vi "Main.vi"(11 "Module Admin":refnum<class "Delacor_lib_QMH_Module Admin.lvclass">) -> ()   [LabVIEW 2025, in "Dashboard.lvlib"]
doc: "This template is based off of the Queued Message Handler design pattern and the Queued Message Handler project template that ships with LabVIEW.\n\nThe main difference is that the queue is private to this module and communication between modules is performed via Broadcast and Request events.\n\nRequest events are wrapped in public API methods and are handled in the Event Handling Loop (EHL) of this VI. Any module can register for Broadcast events sent by this module. The EHL generates messages based on user interface actions.\n\nThe Message Handling Loop (MHL) processes messages generated by the EHL, or by other messages. The messages are string values, so new messages can be added easily to the Message Cases case structure in the MHL. Each message cluster can also provide an optional value for Message Data, which is a variant that can be converted to whatever message-specific data is required.\n_____\nBased on DQMH Dev Tools: Project Template 7.1.2.1547."
uses:
  Dashboard.lvlib
  <vilib>/Delacor/Delacor QMH/Libraries/Module Admin_class/Delacor_lib_QMH_Module Admin.lvclass
  OpCore/SQLite/SQLite.lvclass
  <vilib>/Delacor/Delacor QMH/Libraries/Message Queue_class/Delacor_lib_QMH_Message Queue.lvclass/Delacor_lib_QMH_Message Queue.ctl
  <vilib>/Delacor/Delacor QMH/Libraries/Module Admin_class/Delacor_lib_QMH_Module Admin.lvclass/Delacor_lib_QMH_Module Admin.ctl
  <vilib>/Delacor/Delacor QMH/Libraries/Message Queue_class/Delacor_lib_QMH_Message Queue.lvclass
  Module Data--cluster.ctl
  <vilib>/Utility/miscctls.llb/LVPointTypeDef.ctl
  <vilib>/Delacor/Delacor QMH/Libraries/Message Queue_class/Delacor_lib_QMH_Enqueue Message (Single).vi
  Stop Argument--cluster.ctl
  OpCore/OpCore Types/BaselineMode.ctl
  OpCore/OpCore Types/OpCore Types.lvlib
  OpCore/OpCore Types/Baseline Config.ctl
  OpCore/OpCore Types/ShutdownReason.ctl
  OpCore/OpCore Types/SyncDirection.ctl
  OpCore/OpCore Types/TableOverride.ctl
  OpCore/OpCore Types/StationConfig.ctl
  OpCore/Libraries/Connection Monitor/Connection Monitor.lvlib
  OpCore/Libraries/Inbound Sync/Inbound Sync.lvlib
  OpCore/Libraries/Outbound Sync/Outbound Sync.lvlib
  OpCore/Libraries/Connection Monitor/Database Status.ctl
  OpCore/PostgreSQL/PostgreSQL.lvclass
  Launch Modules Argument--cluster.ctl
  OpCore/OpCore Types/CycleDirection.ctl
  OpCore/OpCore Types/CycleStatus.ctl
  OpCore/OpCore Types/SyncCycleResult.ctl
panel:
  in  "Start":bool
  out "Time Stamp":timestamp
  out "Connected":bool
  out "Online":bool
  in  "Force In Sync":bool
  out "Halt?":bool
  out "Last In Sync Results":T1
  out "Last Out Sync Results":T1
  in  "Force Out Sync":bool
  in  "Start Sync":bool
  in  "stop":bool
  out "Schema Version":string
  out "Station ID":string
  out "error out":errorcluster
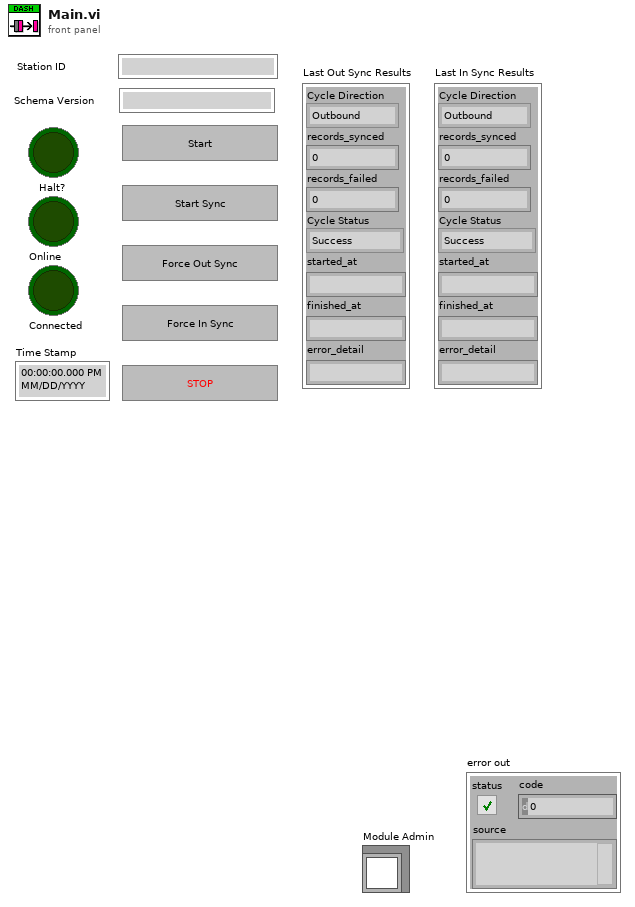
[diagram p1: front panel]
types:
  T1 = typedef "OpCore Types.lvlib/SyncCycleResult.ctl" = cluster{"Cycle Direction":T2, "records_synced":i32, "records_failed":i32, "Cycle Status":T3, "started_at":string, "finished_at":string, "error_detail":string}
  T2 = typedef "OpCore Types.lvlib/CycleDirection.ctl" = enum16{"Outbound", "Inbound", "Startup", "Shutdown", "Baseline", "Provision", "Migration", "Config"}
  T3 = typedef "OpCore Types.lvlib/CycleStatus.ctl" = enum16{"Success", "Partial", "Failed"}
  T4 = typedef "Connection Monitor.lvlib/Broadcast Events--cluster.ctl" = cluster{"Module Did Init":refnum<user-event>, "Status Updated":refnum<user-event>, "Error Reported":refnum<user-event>, "Module Did Stop":refnum<user-event>, "Update Module Execution Status":refnum<user-event>, "Database Online":refnum<user-event>, "Database Offline":refnum<user-event>, "Database Status Updated":refnum<user-event>}
  T5 = typedef "Outbound Sync.lvlib/Broadcast Events--cluster.ctl" = cluster{"Module Did Init":refnum<user-event>, "Status Updated":refnum<user-event>, "Error Reported":refnum<user-event>, "Module Did Stop":refnum<user-event>, "Update Module Execution Status":refnum<user-event>, "Sync Completed":refnum<user-event>}
  T6 = typedef "Inbound Sync.lvlib/Broadcast Events--cluster.ctl" = cluster{"Module Did Init":refnum<user-event>, "Status Updated":refnum<user-event>, "Error Reported":refnum<user-event>, "Module Did Stop":refnum<user-event>, "Update Module Execution Status":refnum<user-event>, "Sync Completed":refnum<user-event>}
  T7 = typedef "Dashboard.lvlib/Request Events--cluster.ctl" = cluster{"Stop Module":refnum<user-event>, "Show Panel":refnum<user-event>, "Hide Panel":refnum<user-event>, "Get Module Execution Status":refnum<user-event>, "Show Diagram":refnum<user-event>, "Private.Launch Modules":refnum<user-event>}
  T8 = typedef "Dashboard.lvlib/Module Data--cluster.ctl" = cluster{"Status":string, "SQLite":refnum<class "SQLite.lvclass">, "StationConfig":T9, "OB Module ID":i32, "IB Module ID":i32, "is online":bool, "CM alive?":bool, "OB alive?":bool, "IB alive?":bool, "IB first cycle seen?":bool, "OB first cycle seen?":bool, "shutting down?":bool, "exit code":i32, "status":bool, "code":i32, "source":string, "ShutdownReason":T12, "OB last cycle at":timestamp, "IB last cycle at":timestamp, "Baseline Config":T13}
  T9 = typedef "OpCore Types.lvlib/StationConfig.ctl" = cluster{"station_id":string, "schema_version":string, "sqlite_path":string, "syncagent_db_path":string, "postgres_conn":string, "sync_interval_sec":i32, "inbound_offset_sec":i32, "batch_size":i32, "table_overrides":T10[]}
  T10 = typedef "OpCore Types.lvlib/TableOverride.ctl" = cluster{"table_name":string, "Sync Direction":T11}
  T11 = typedef "OpCore Types.lvlib/SyncDirection.ctl" = enum16{"Both", "Outbound_Only", "Inbound_Only", "Exclude"}
  T12 = typedef "OpCore Types.lvlib/ShutdownReason.ctl" = enum16{"None", "Operator", "Service", "ModuleDied", "Fatal"}
  T13 = typedef "OpCore Types.lvlib/Baseline Config.ctl" = cluster{"Baseline Mode":T14, "From Date":string, "Chunk Size":i32, "Verify Checksums":bool}
  T14 = typedef "OpCore Types.lvlib/BaselineMode.ctl" = enum16{"None", "Full", "From Date"}
  T15 = enum32{"invalid lock state", "Not Locked", "Locked (No Password)", "Password-protected"}
  T16 = typedef "Dashboard.lvlib/Stop Argument--cluster.ctl" = cluster{"Origin":string, "Exit via Stop Module Req?":bool, "Wait for Module to stop?":bool}
  T17 = typedef "Connection Monitor.lvlib/Database Status.ctl" = cluster{"Time Stamp":timestamp, "isOnline?":bool}
  T18 = typedef "Dashboard.lvlib/Launch Modules Argument--cluster.ctl" = cluster{"OB Module ID":i32, "IB Module ID":i32}
  T19 = typedef "LVPointTypeDef.ctl" = cluster{"Horizontal":i16, "Vertical":i16}
  T20 = enum32{"Invalid", "Standard", "Closed", "Hidden", "Minimized", "Maximized"}
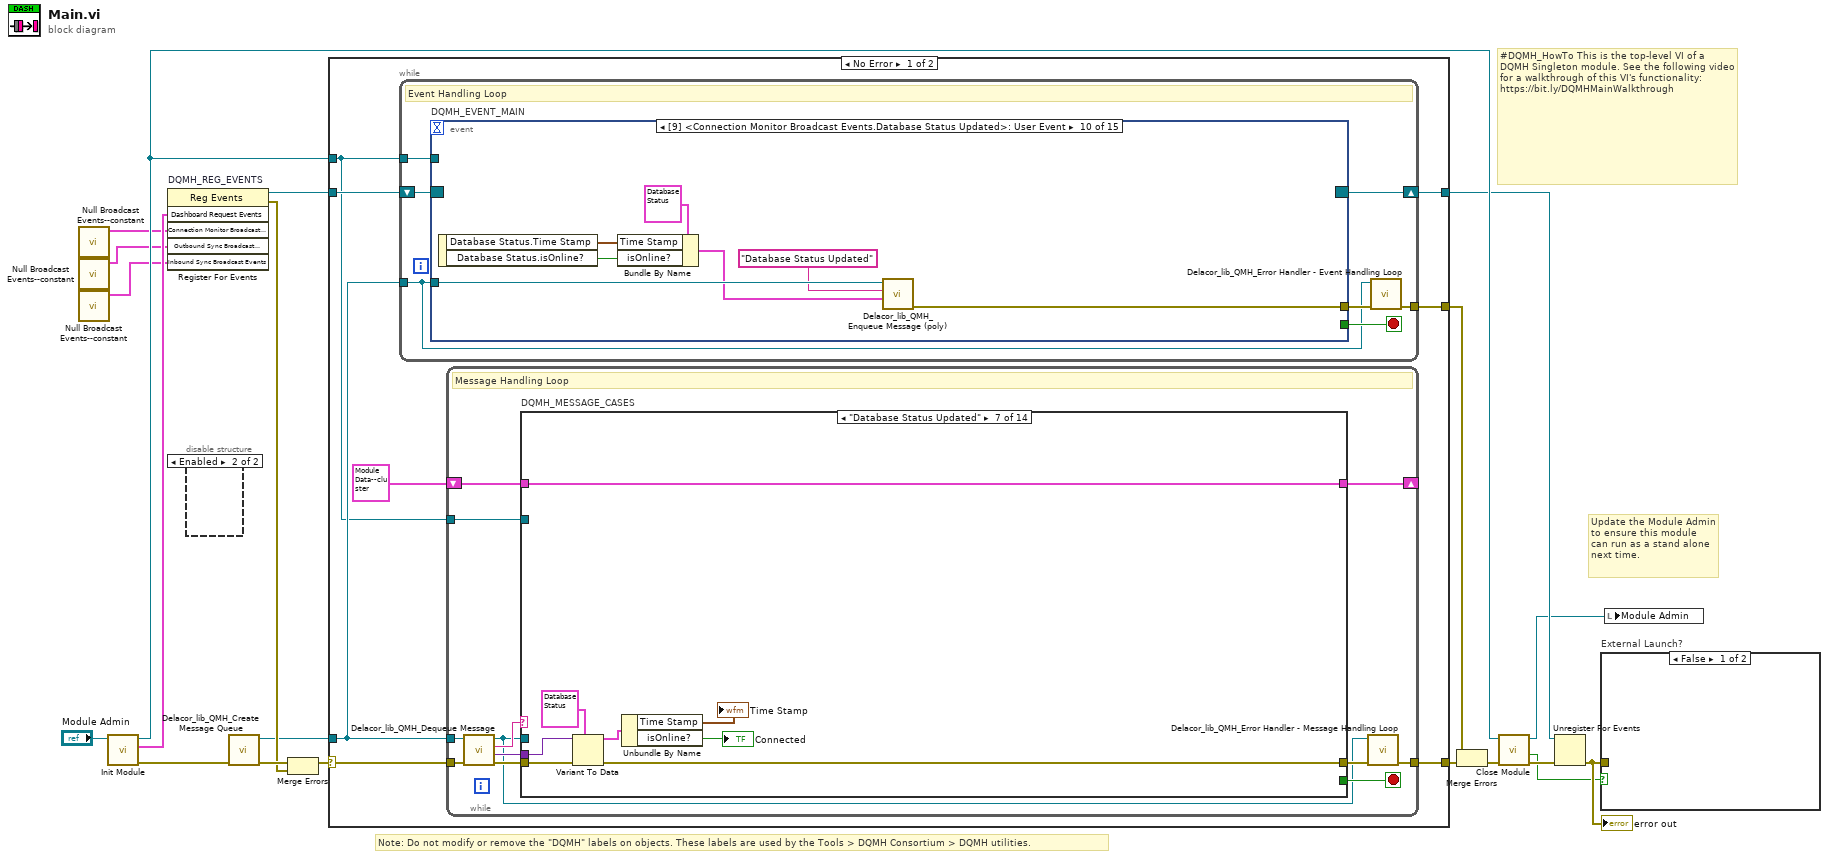
[diagram p0: block diagram]
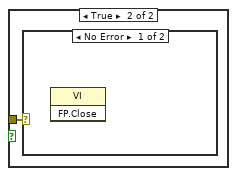
[diagram p3: hidden frame]
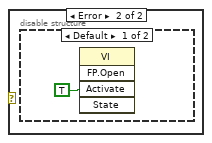
[diagram p4: hidden frame]
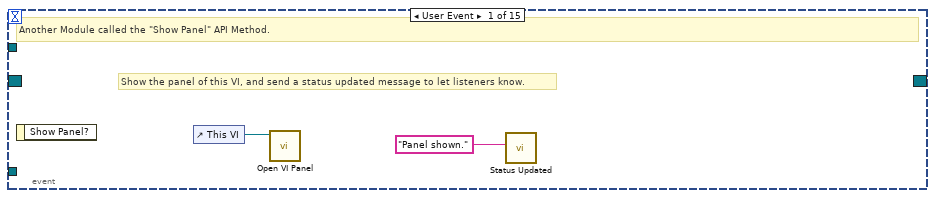
[diagram p6: hidden frame]
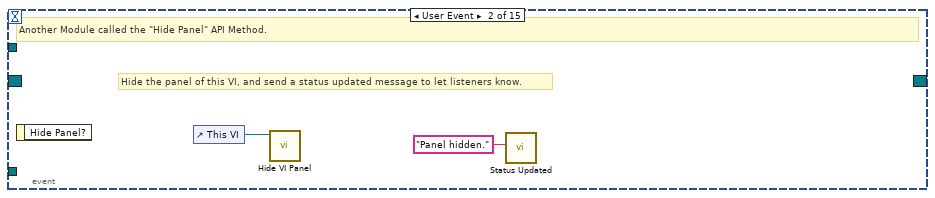
[diagram p7: hidden frame]
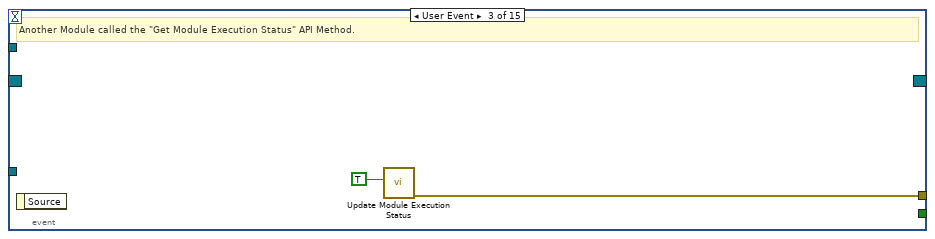
[diagram p8: hidden frame]
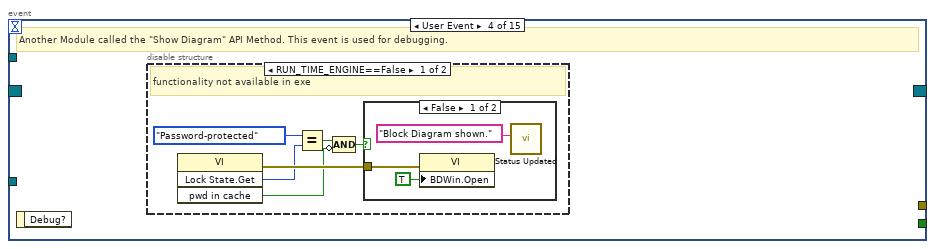
[diagram p9: hidden frame]
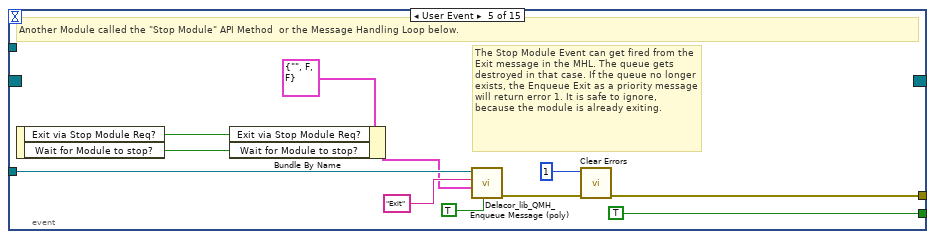
[diagram p12: hidden frame]
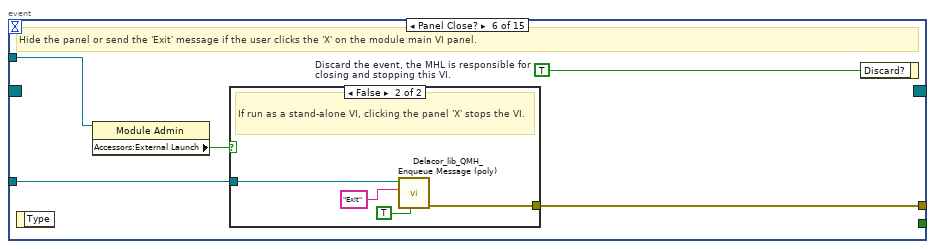
[diagram p13: hidden frame]
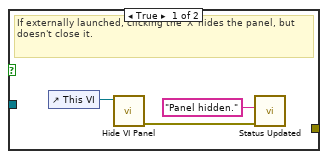
[diagram p14: hidden frame]
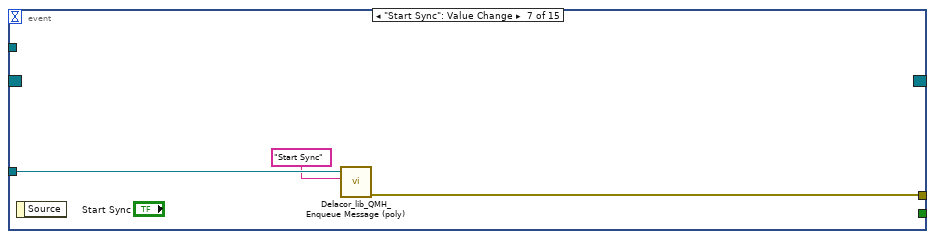
[diagram p15: hidden frame]
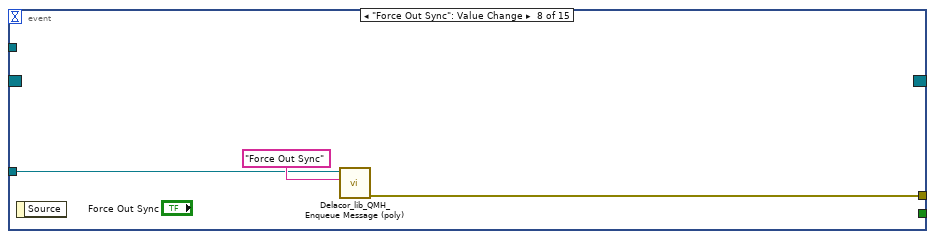
[diagram p16: hidden frame]
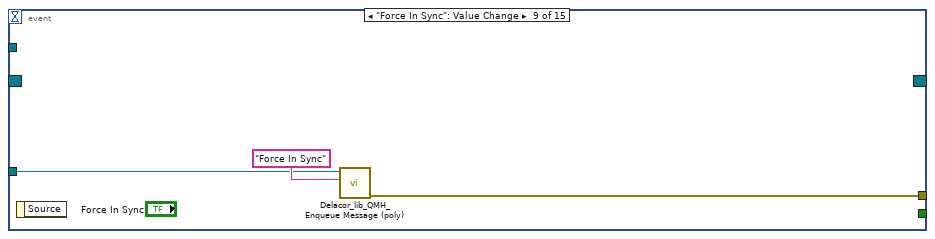
[diagram p17: hidden frame]
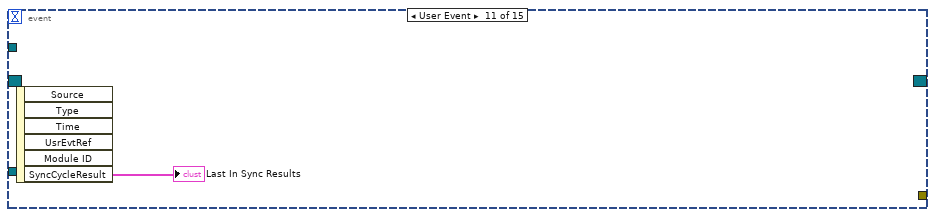
[diagram p18: hidden frame]
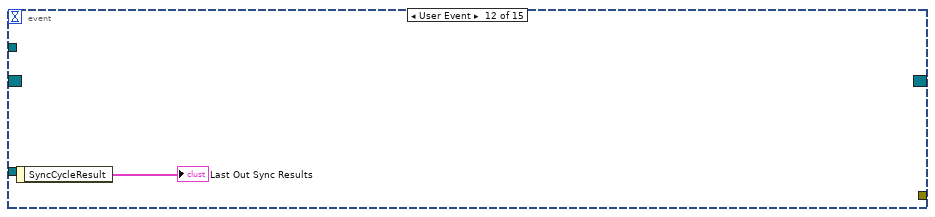
[diagram p19: hidden frame]
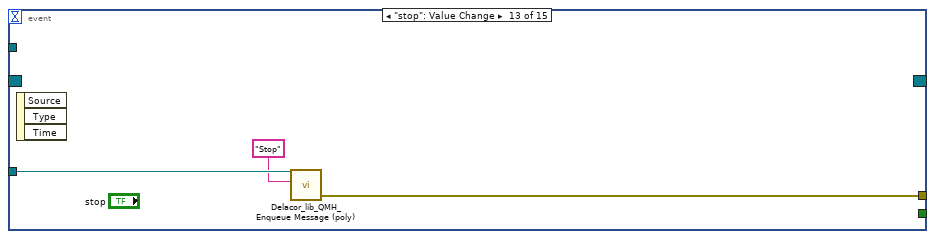
[diagram p20: hidden frame]
diagram:
  # "#DQMH_HowTo This is the top-level VI of a DQMH Singleton module. See the following video for a walkthrough of this VI's functionality: https://bit.ly/DQMHMainWalkthrough"
  # "Note: Do not modify or remove the \"DQMH\" labels on objects. These labels are used by the Tools > DQMH Consortium > DQMH utilities."
  # "Update the Module Admin to ensure this module can run as a stand alone next time."
  n1 = call "Null Broadcast Events--constant.vi"() -> ("Connection Monitor Broadcast Events"=w3:T4)  [unwired: 11 in]
  n2 = call "Null Broadcast Events--constant.vi"() -> ("Outbound Sync Broadcast Events"=w2:T5)  [unwired: 11 in]
  n3 = call "Null Broadcast Events--constant.vi"() -> ("Inbound Sync Broadcast Events"=w1:T6)  [unwired: 11 in]
  n4 = call "Init Module.vi"("Singleton Module Admin in"="Module Admin") -> ("error out"=w19:errorcluster, "Dashboard Request Events"=w8:T7, "Singleton Module Admin out"=w11:refnum<class "Delacor_lib_QMH_Module Admin.lvclass">)  [unwired: 8 in]
  n5 = register-events "DQMH_REG_EVENTS"(w8, w3, w2, w1) -> (reference out=w9:refnum<event-registration>, error out=w12:errorcluster)  [unwired: 2 in]
  n6 = disable-structure shown="Enabled" {
    frame Disabled {
    }
    frame Enabled {
    }
  }
  n7 = call <vilib>:"Delacor_lib_QMH_Create Message Queue.vi"("error in"=w19) -> ("error out"=w14:errorcluster, "Message Queue"=w7:refnum<class "Delacor_lib_QMH_Message Queue.lvclass">)  [unwired: 9 in]
  n8 = Merge Errors(w14, w12) -> (w13:errorcluster)
  n9 = case shown="No Error" w13 {
    selector: w13 -> [w26 w268]
    tunnel: [w28 w267] -> w20
    tunnel: [w25 w266] -> w10
    tunnel: w9 -> [w23 w266]
    tunnel: w7 -> [w22 w261]
    tunnel: [w27 _] -> w17
    tunnel: w11 -> [w21 w262]
    frame No Error {
      n10 = while {
        tunnel: w22 -> [w29]
        shift-right: [w32] -> w25
        shift-left: w23 -> [w33]
        tunnel: [w34] -> w27
        tunnel: w21 -> [w30]
        stop <- w31 stop-if-true
        # "Event Handling Loop"
        n11 = event "DQMH_EVENT_MAIN" shown="[9] <Connection Monitor Broadcast Events.Database Status Updated>: User Event" {
          selector: w33 -> [_ _ _ _ _ _ _ _ _ _ _ _ _ _ w110]
          dyn-events: [_ _ _ _ _ _ _ _ _ _ _ _ _ _ w106] -> w32
          timeout: _ -> [_ _ _ _ _ _ _ _ _ _ _ _ _ _ _]
          tunnel: [_ _ _ _ TRUE ("Discard?") _ _ _ _ _ _ _ _ _ _] -> w31
          tunnel: w29 -> [_ _ _ _ w57 w64 w76 w77 w80 w89 _ _ w94 w101 _]
          tunnel: [_ _ w41 _ w60 w66 w74 w78 w81 w88 _ _ w93 w95 w102] -> w35
          tunnel: w30 -> [_ _ _ _ _ w63 _ _ _ _ _ _ _ _ _]
          event User Event {
            # "Show the panel of this VI, and send a status updated message to let listeners know."
            # "Another Module called the \"Show Panel\" API Method."
            n12 = event-data() -> ()  [unwired: 1 in, 1 out]
            n13 = control-ref of="This VI"() -> (w37:refnum<vi>)
            n14 = call "Open VI Panel.vi"("VI"=w37) -> ()  [unwired: 10 in, 1 out]
            n15 = call "Status Updated.vi"("Status"="Panel shown." ("format string")) -> ()  [unwired: 10 in, 1 out]
          }
          event User Event {
            # "Hide the panel of this VI, and send a status updated message to let listeners know."
            # "Another Module called the \"Hide Panel\" API Method."
            n16 = event-data() -> ()  [unwired: 1 in, 1 out]
            n17 = control-ref of="This VI"() -> (w39:refnum<vi>)
            n18 = call "Hide VI Panel.vi"("VI"=w39) -> ()  [unwired: 10 in, 1 out]
            n19 = call "Status Updated.vi"("Status"="Panel hidden." ("format string")) -> ()  [unwired: 10 in, 1 out]
          }
          event User Event {
            # "Another Module called the \"Get Module Execution Status\" API Method."
            n20 = event-data() -> ()  [unwired: 1 in, 1 out]
            n21 = call "Update Module Execution Status.vi"("Running?"=TRUE) -> ("error out"=w41:errorcluster)  [unwired: 10 in]
          }
          event User Event {
            # "Another Module called the \"Show Diagram\" API Method. This event is used for debugging."
            n22 = event-data() -> ()  [unwired: 1 in, 1 out]
            n23 = disable-structure shown="RUN_TIME_ENGINE==False" {
              frame condition #0 (active) {
                # "functionality not available in exe"
                n24 = invoke on="Invoke Node" class="VI" method="Lock State.Get"() -> (error out=w47:errorcluster, "Get Lock State"=w46:T15, "pwd in cache"=w43:bool)  [unwired: 4 in, 1 out]
                n25 = Equal?(x=T15."Password-protected", y=w46) -> (x = y?=w44:bool)
                n26 = Compound Arithmetic op=AND(w44, invert w43) -> (w42:bool)
                n27 = case shown="False" w42 {
                  tunnel: w47 -> [w50 _]
                  frame False {
                    n28 = property on="Property Node" class="VI"(error in=w50, "BDWin.Open"=TRUE ("Block Diagram Window:Open")) -> ()  [unwired: 1 in, 2 out]
                    n29 = call "Status Updated.vi"("Status"="Block Diagram shown." ("format string")) -> ()  [unwired: 10 in, 1 out]
                  }
                  frame True {
                    # "Password-protected VI, and the password is not in the cache. Do not show the diagram."
                  }
                }
              }
              frame condition #1 {
              }
            }
          }
          event User Event {
            # "The Stop Module Event can get fired from the Exit message in the MHL. The queue gets destroyed in that case. If the queue no longer exists, the Enqueue Exit as a priority message will return error 1. It is safe to ignore, because the module is already exiting."
            # "Another Module called the \"Stop Module\" API Method  or the Message Handling Loop below."
            n30 = event-data() -> ("Exit via Stop Module Req?"=w53:bool, "Wait for Module to stop?"=w52:bool)  [unwired: 1 in]
            n31 = Bundle By Name(cluster=T16 {"Origin"="", "Exit via Stop Module Req?"=FALSE, "Wait for Module to stop?"=FALSE} ("Stop Argument"), "Exit via Stop Module Req?"=w53, "Wait for Module to stop?"=w52) -> (w51:T16)
            n32 = call-poly <vilib>:"Delacor_lib_QMH_Enqueue Message (poly).vi"("Priority Message? (F)"=TRUE, "Message Data"=w51, "Message"="Exit", "Message Queue in"=w57) -> ("error out"=w61:errorcluster)  [unwired: 6 in, 1 out]
            n33 = call <vilib>:"Clear Errors.vi"("error in (no error)"=w61, "specific error code to clear (0: all)"=1) -> ("error out"=w60:errorcluster)  [unwired: 4 in, 1 out]
          }
          event Panel Close? {
            w65 = TRUE  # Discard the event, the MHL is responsible for closing and stopping this VI.
            # "Hide the panel or send the 'Exit' message if the user clicks the 'X' on the module main VI panel."
            n34 = event-data() -> ()  [unwired: 1 in, 1 out]
            n35 = property on="Property Node" class="Module Admin"(reference=w63) -> ("Accessors:External Launch"=w62:bool)  [unwired: 1 in, 2 out]
            n36 = case shown="False" w62 {
              tunnel: w64 -> [_ w72]
              tunnel: [_ w73] -> w66
              frame True {
                # "If externally launched, clicking the 'X' hides the panel, but doesn't close it."
                n37 = control-ref of="This VI"() -> (w69:refnum<vi>)
                n38 = call "Hide VI Panel.vi"("VI"=w69) -> ("error out"=w67:errorcluster)  [unwired: 10 in]
                n39 = call "Status Updated.vi"("error in"=w67, "Status"="Panel hidden." ("format string")) -> ()  [unwired: 9 in, 1 out]
              }
              frame False {
                # "If run as a stand-alone VI, clicking the panel 'X' stops the VI."
                n40 = call-poly <vilib>:"Delacor_lib_QMH_Enqueue Message (poly).vi"("Priority Message? (F)"=TRUE, "Message"="Exit", "Message Queue in"=w72) -> ("error out"=w73:errorcluster)  [unwired: 7 in, 1 out]
              }
            }
            n41 = event-data ("Event Filter Node")("Discard?"=w65) -> ()  [unwired: 1 in, 1 out]
          }
          event "Start Sync": Value Change {
            n42 = event-data() -> ()  [unwired: 1 in, 1 out]
            n43 = call-poly <vilib>:"Delacor_lib_QMH_Enqueue Message (poly).vi"("Message"="Start Sync", "Message Queue in"=w76) -> ("error out"=w74:errorcluster)  [unwired: 8 in, 1 out]
          }
          event "Force Out Sync": Value Change {
            n44 = event-data() -> ()  [unwired: 1 in, 1 out]
            n45 = call-poly <vilib>:"Delacor_lib_QMH_Enqueue Message (poly).vi"("Message"="Force Out Sync", "Message Queue in"=w77) -> ("error out"=w78:errorcluster)  [unwired: 8 in, 1 out]
          }
          event "Force In Sync": Value Change {
            n46 = event-data() -> ()  [unwired: 1 in, 1 out]
            n47 = call-poly <vilib>:"Delacor_lib_QMH_Enqueue Message (poly).vi"("Message"="Force In Sync", "Message Queue in"=w80) -> ("error out"=w81:errorcluster)  [unwired: 8 in, 1 out]
          }
          event User Event {
            n48 = event-data() -> ("Database Status.Time Stamp"=w87:timestamp, "Database Status.isOnline?"=w85:bool)  [unwired: 1 in]
            n49 = Bundle By Name(cluster=T17 {"Time Stamp"=timestamp(0 s since 1904-01-01), "isOnline?"=FALSE} ("Database Status"), "Time Stamp"=w87, "isOnline?"=w85) -> (w84:T17)
            n50 = call-poly <vilib>:"Delacor_lib_QMH_Enqueue Message (poly).vi"("Message Data"=w84, "Message"="Database Status Updated", "Message Queue in"=w89) -> ("error out"=w88:errorcluster)  [unwired: 7 in, 1 out]
          }
          event User Event {
            n51 = event-data() -> ("SyncCycleResult"=→"Last In Sync Results":T1)  [unwired: 1 in, 5 out]
          }
          event User Event {
            n52 = event-data() -> ("SyncCycleResult"=→"Last Out Sync Results":T1)  [unwired: 1 in]
          }
          event "stop": Value Change {
            n53 = event-data() -> ()  [unwired: 1 in, 3 out]
            n54 = call-poly <vilib>:"Delacor_lib_QMH_Enqueue Message (poly).vi"("Message"="Stop", "Message Queue in"=w94) -> ("error out"=w93:errorcluster)  [unwired: 8 in, 1 out]
          }
          event User Event {
            # "This module called the \"Private.Launch Modules\" private request."
            n55 = event-data() -> ("OB Module ID"=w97:i32, "IB Module ID"=w96:i32)  [unwired: 1 in]
            n56 = Bundle(cluster=T18 {"OB Module ID"=-1, "IB Module ID"=-1} ("Launch Modules Argument"), "OB Module ID"=w97, "IB Module ID"=w96) -> (w98:T18)
            n57 = call-poly <vilib>:"Delacor_lib_QMH_Enqueue Message (poly).vi"("Message Data"=w98, "Message"="Launch Modules", "Message Queue in"=w101) -> ("error out"=w95:errorcluster)  [unwired: 7 in, 1 out]
          }
          event "Start": Value Change {
            n58 = event-data() -> ()  [unwired: 1 in, 1 out]
            n59 = call "Start Module.vi"() -> ("error out"=w120:errorcluster, "Wait for Event Sync?"=w117:bool, "Connection Monitor Broadcast Events"=w109:T4)  [unwired: 7 in, 2 out]
            n60 = call "Synchronize Module Events.vi"("error in"=w120, "Wait for Event Sync?"=w117) -> ("error out"=w112:errorcluster)  [unwired: 9 in]
            n61 = call "Start Module.vi"("error in"=w112) -> ("error out"=w119:errorcluster, "Wait for Event Sync?"=w116:bool, "Outbound Sync Broadcast Events"=w108:T5, "Module ID"=w114:i32)  [unwired: 6 in, 1 out]
            n62 = call "Synchronize Module Events.vi"("error in"=w119, "Wait for Event Sync?"=w116, "Module ID in"=w114) -> ("error out"=w111:errorcluster, "Module ID out"=w103:i32)  [unwired: 7 in]
            n63 = call "Start Module.vi"("error in"=w111) -> ("error out"=w118:errorcluster, "Wait for Event Sync?"=w115:bool, "Inbound Sync Broadcast Events"=w107:T6, "Module ID"=w113:i32)  [unwired: 6 in, 1 out]
            n64 = call "Synchronize Module Events.vi"("error in"=w118, "Wait for Event Sync?"=w115, "Module ID in"=w113) -> ("error out"=w105:errorcluster, "Module ID out"=w104:i32)  [unwired: 7 in]
            n65 = register-events ("DQMH_REG_EVENTS")(reference=w110, w109, w108, w107) -> (reference out=w106:refnum<event-registration>)  [unwired: 2 in, 1 out]
            n66 = call "Launch Modules.vi"("error in"=w105, "IB Module ID"=w104, "OB Module ID"=w103) -> ("error out"=w102:errorcluster)  [unwired: 8 in]
          }
        }
        n67 = call-dynamic "Delacor_lib_QMH_Error Handler - Event Handling Loop.vi"("error in"=w35, "Message Queue in"=w29) -> ("dup error in"=w34:errorcluster)  [unwired: 8 in, 1 out]
      }
      n68 = while {
        tunnel: w22 -> [w121]
        shift-right: [w129] -> _
        shift-left: T8 {"Status"="", "SQLite"=refnum, "StationConfig"={"station_id"="", "schema_version"="", "sqlite_path"="", "syncagent_db_path"="", "postgres_conn"="", "sync_interval_sec"=0, "inbound_offset_sec"=0, "batch_size"=0, "table_overrides"=[]}, "OB Module ID"=-1, "IB Module ID"=-1, "is online"=FALSE, "CM alive?"=FALSE, "OB alive?"=FALSE, "IB alive?"=FALSE, "IB first cycle seen?"=FALSE, "OB first cycle seen?"=FALSE, "shutting down?"=FALSE, "exit code"=0, "status"=FALSE, "code"=0, "source"="", "ShutdownReason"=enum."None", "OB last cycle at"=timestamp(0 s since 1904-01-01), "IB last cycle at"=timestamp(0 s since 1904-01-01), "Baseline Config"={"Baseline Mode"=enum."None", "From Date"="", "Chunk Size"=1000, "Verify Checksums"=TRUE}} ("Data Cluster") -> [w130]
        tunnel: w26 -> [w132]
        tunnel: [w124] -> w28
        tunnel: w21 -> [w125]
        stop <- w128 stop-if-true
        # "Message Handling Loop"
        n69 = call-dynamic "Delacor_lib_QMH_Dequeue Message.vi"("error in"=w132, "Message Queue in"=w121) -> ("error out"=w131:errorcluster, "Message Data"=w126:variant, "Message"=w127:string, "Message Queue out"=w122:refnum<class "Delacor_lib_QMH_Message Queue.lvclass">)  [unwired: 6 in]
        n70 = case "DQMH_MESSAGE_CASES" shown="\"Database Status Updated\"" w127 {
          selector: w127 -> [_ _ _ _ _ _ _ _ _ _ _ _ _ w256]
          tunnel: w122 -> [_ _ _ _ _ _ _ _ _ _ _ w222 w244 _]
          tunnel: w131 -> [w157 w167 w169 w177 w178 w186 w194 w196 w213 w216 w218 w229 w250 w259]
          tunnel: [w156 w167 w169 w176 w179 w187 w193 w197 w212 w215 w218 w225 w245 w260] -> w123
          tunnel: w130 -> [w143 w166 w168 w173 w181 w184 w195 w204 w207 w214 w217 w224 w243 w257]
          tunnel: [w137 w166 w168 w173 w181 w184 w195 w204 w205 w214 w217 w224 w243 w257] -> w129
          tunnel: [_ _ _ _ _ _ _ _ _ _ _ _ w242 _] -> w128
          tunnel: w126 -> [_ _ _ _ _ _ w192 _ w211 _ _ w223 w241 _]
          tunnel: w125 -> [w148 _ _ _ _ _ _ _ _ _ _ w221 w236 _]
          frame "Initialize" {
            # "Initialize - Any operation that needs to be done before the module can receive messages. Synchronize Caller Events.vi will inform Start Module.vi that the module has launched and is ready to receive messages. Module Did Init.vi will broadcast that the module initialized."
            n71 = call "Synchronize Caller Events.vi"("error in"=w157, "Singleton Module Admin in"=w148) -> ("error out"=w142:errorcluster, "Singleton Module Admin out"=w145:refnum<class "Delacor_lib_QMH_Module Admin.lvclass">)  [unwired: 8 in]
            n72 = property on="Property Node" class="Module Admin"(reference=w145) -> ("Accessors:External Launch"=w152:bool)  [unwired: 1 in, 2 out]
            n73 = call "Module Name--constant.vi"() -> ("Module Name"=w155:string)  [unwired: 11 in]
            n74 = property on="Property Node" class="VI"("Front Panel.Title"=w155) -> (reference out=w154:refnum<vi>, error out=w159:errorcluster)  [unwired: 2 in]
            n75 = Select(t=T20."Hidden" ("State"), s=w152, f=T20."Standard" ("State")) -> (s? t:f=w149:T20)
            n76 = invoke on="Invoke Node" class="VI" method="FP.Open"(reference=w154, error in=w159, "State"=w149) -> (reference out=w153:refnum<vi>, error out=w158:errorcluster)  [unwired: 2 in, 3 out]
            n77 = property on="Pane" class="Pane"("Origin"=T19 {"Horizontal"=0, "Vertical"=0}) -> ()  [unwired: 2 in, 2 out]
            n78 = invoke on="Invoke Node" class="VI" method="FP.Center"(reference=w153, error in=w158) -> ()  [unwired: 1 in, 3 out]
            n79 = disable-structure shown="Enabled" {
              disable-tunnel: w143 -> [w163 w164]
              disable-tunnel: w142 -> [w162 w165]
              disable-tunnel: [w161 w165] -> w141
              disable-tunnel: [w160 w164] -> w139
              frame Disabled {
                n80 = call "Launch.vi"("error in (no error)"=w162, "Data Cluster In"=w163) -> ("error out"=w161:errorcluster, "Data Cluster Out"=w160:T8)  [unwired: 8 in]
              }
              frame Enabled {
              }
            }
            n81 = call "Startup.vi"("error in (no error)"=w141, "Data Cluster In"=w139) -> ("error out"=w140:errorcluster, "halt?"=→"Halt?":bool, "Data Cluster Out"=w137:T8)  [unwired: 7 in]
            n82 = Unbundle By Name(w137) -> ("StationConfig.station_id"=→"Station ID":string, "StationConfig.schema_version"=→"Schema Version":string, "StationConfig.postgres_conn"=w134:string)
            n83 = call "Ping.vi"("Connection String"=w134) -> ("is_Online"=→"Online":bool)  [unwired: 9 in, 1 out]
            n84 = call "Module Name--constant.vi"() -> ("Module Name"=w146:string)  [unwired: 11 in]
            n85 = call "Module Did Init.vi"("error in"=w140, "Initialized?"=TRUE, "Origin"=w146) -> ("error out"=w156:errorcluster)  [unwired: 8 in]
          }
          frame "---Module Specific---" {
            # "Separator -- The following cases handle messages specific to this Module."
          }
          frame "Start" {
          }
          frame "Start Sync" {
            n86 = Unbundle By Name(w173) -> ("OB Module ID"=w170:i32, "IB Module ID"=w171:i32, "StationConfig"=w172:T9)
            n87 = call "Start Outbound Sync.vi"("StationConfig"=w172, "Module ID"=w170) -> ("error out"=w175:errorcluster)  [unwired: 9 in]
            n88 = call "Start Inbound Sync.vi"("StationConfig"=w172, "Module ID"=w171) -> ("error out"=w174:errorcluster)  [unwired: 9 in]
            n89 = Merge Errors(w177, w175, w174) -> (w176:errorcluster)
          }
          frame "Force Out Sync" {
            n90 = Unbundle By Name(w181) -> ("OB Module ID"=w180:i32)
            n91 = call "Force Sync.vi"("error in"=w178, "Force Sync"=TRUE, "Module ID"=w180) -> ("error out"=w179:errorcluster)  [unwired: 8 in]
          }
          frame "Force In Sync" {
            n92 = Unbundle By Name(w184) -> ("IB Module ID"=w183:i32)
            n93 = call "Force Sync.vi"("error in"=w186, "Force Sync"=TRUE, "Module ID"=w183) -> ("error out"=w187:errorcluster)  [unwired: 8 in]
          }
          frame "Database Status Updated" {
            n94 = Variant To Data(error in=w194, type=T17 {"Time Stamp"=timestamp(0 s since 1904-01-01), "isOnline?"=FALSE} ("Database Status"), Variant=w192) -> (data=w190:T17, error out=w193:errorcluster)
            n95 = Unbundle By Name(w190) -> ("Time Stamp"=→"Time Stamp":timestamp, "isOnline?"=→"Connected":bool)
          }
          frame "Stop" {
            w201 = TRUE ("Wait for Module to Stop? (F)")
            n96 = Unbundle By Name(w204) -> ("IB Module ID"=w203:i32, "OB Module ID"=w202:i32)
            n97 = call "Stop Module.vi"("Wait for Module to Stop? (F)"=w201) -> ("error out"=w200:errorcluster)  [unwired: 10 in]
            n98 = call "Stop Module.vi"("Wait for Module to stop? (F)"=w201, "Module ID"=w203) -> ("error out"=w199:errorcluster)  [unwired: 9 in]
            n99 = call "Stop Module.vi"("Wait for Module to stop? (F)"=w201, "Module ID"=w202) -> ("error out"=w198:errorcluster)  [unwired: 9 in]
            n100 = Merge Errors(w196, w200, w199, w198) -> (w197:errorcluster)
          }
          frame "Launch Modules" {
            n101 = Variant To Data(error in=w213, type=T18 {"OB Module ID"=-1, "IB Module ID"=-1} ("Launch Modules Argument"), Variant=w211) -> (data=w209:T18, error out=w212:errorcluster)
            n102 = Unbundle By Name(w209) -> ("OB Module ID"=w208:i32, "IB Module ID"=w206:i32)
            n103 = Bundle By Name(cluster=w207, "OB Module ID"=w208, "IB Module ID"=w206) -> (w205:T8)
          }
          frame "---Copy This Frame---" {
            # "Duplicate this frame when creating new messages.  Change this comment in the duplicated frame to describe this message."
            n104 = Merge Errors(w216) -> (w215:errorcluster)
          }
          frame "---Exit and Error Handling---" {
            # "Separator - The following cases handle errors and exit messages."
          }
          frame "Error" {
            # "#DQMH_CodeRecommended - If the module is running in standalone mode (External Launch = FALSE), this code will pop up an error dialog and call the 'Exit' message if an error occurs. Add more fine-grained error management here."
            # "Error - Check the error message data and respond accordingly. This message is sent by the \"Error Handler\" VIs at the end of each loop in this application."
            n105 = property on="Property Node" class="Module Admin"(reference=w221) -> ("Accessors:External Launch"=w220:bool)  [unwired: 1 in, 2 out]
            n106 = Variant To Data(error in=w229, type=errorcluster {"status"=FALSE, "code"=0, "source"=""} ("error constant"), Variant=w223) -> (data=w219:errorcluster, error out=w227:errorcluster)
            n107 = local write "error out"(w219) -> ()
            n108 = call "Error Reported.vi"("Error"=w219) -> ()  [unwired: 10 in, 1 out]
            n109 = case shown="False" w220 {
              tunnel: [w234 _] -> w226
              tunnel: w222 -> [w232 _]
              tunnel: w219 -> [w233 _]
              frame False {
                n110 = disable-structure shown="Default" {
                  disable-tunnel: w233 -> [w235 _]
                  frame condition #0 (active) {
                    # "If the module is running standalone, then pop up an error dialog and call the \"Exit\" message."
                    n111 = call <vilib>:"Simple Error Handler.vi"("error in (no error)"=w235) -> ()  [unwired: 4 in, 5 out]
                  }
                  frame condition #1 {
                    # "To prevent the Simple Error Handler VI from being loaded (e.g. when deploying to a Real-Time target), add the Conditional Disable Symbol \"DQMH_Disable_SEH\" to your project and set it to TRUE."
                  }
                }
                n112 = call-poly <vilib>:"Delacor_lib_QMH_Enqueue Message (poly).vi"("Priority Message? (F)"=TRUE, "Message"="Exit", "Message Queue in"=w232) -> ("error out"=w234:errorcluster)  [unwired: 7 in, 1 out]
              }
              frame True {
                # "If the module was launched externally, calling the Error Reported broadcast VI is the only action performed by the \"Error\" message. The module's caller can then process the error appropriately."
              }
            }
            n113 = Merge Errors(w227, w226) -> (w225:errorcluster)
          }
          frame "Exit" {
            w240 = 91  # 91: not all Exit messages will have an argument
            w242 = TRUE  # Stop the VI
            # "Release the message queue reference"
            # "#DQMH_CodeNeeded - Add any required cleanup code here."
            # "Exit - Exit the application."
            n114 = Variant To Data(error in=w250, type=T16 {"Origin"="", "Exit via Stop Module Req?"=FALSE, "Wait for Module to stop?"=FALSE} ("Stop Argument"), Variant=w241) -> (data=w238:T16, error out=w247:errorcluster)
            n115 = call <vilib>:"Clear Errors.vi"("error in (no error)"=w247, "specific error code to clear (0: all)"=w240) -> ("error out"=w249:errorcluster)  [unwired: 4 in, 1 out]
            n116 = control-ref of="This VI"() -> (w237:refnum<vi>)
            n117 = call-dynamic "Delacor_lib_QMH_Release Message Queue.vi"("error in"=w249, "Message Queue"=w244) -> ("error out"=w248:errorcluster)  [unwired: 9 in]
            n118 = call "Handle Exit.vi"("Stop Argument"=w238, "Admin in"=w236, "VI reference"=w237) -> ("error out"=w246:errorcluster)  [unwired: 7 in, 1 out]
            n119 = Merge Errors(w248, w246) -> (w245:errorcluster)
            n120 = call "Error Reported.vi"("Error"=w245) -> ()  [unwired: 10 in, 1 out]
          }
          frame Default {
            # "'Default' case only runs if there is a message that isn't defined in any of the other cases.  Output a programming error."
            n121 = call "Module Name--constant.vi"() -> ("Module Name"=w255:string)  [unwired: 11 in]
            n122 = Format Into String(format string="The invalid message string \"%s\" was received in the Message Handling Loop for module \"%s\".", w256, w255) -> (resulting string=w251:string)  [unwired: 2 in, 1 out]
            n123 = call <vilib>:"Error Cluster From Error Code.vi"("show call chain? (False)"=TRUE, "error message (\"\")"=w251, "error code (0)"=1) -> ("error out"=w258:errorcluster)  [unwired: 6 in]
            n124 = Merge Errors(w259, w258) -> (w260:errorcluster)
          }
        }
        n125 = call-dynamic "Delacor_lib_QMH_Error Handler - Message Handling Loop.vi"("error in"=w123, "Message Queue in"=w122) -> ("dup error in"=w124:errorcluster)  [unwired: 8 in, 1 out]
      }
    }
    frame Error {
      # "Synchronize Caller Events.vi will inform Start Module.vi that the module has launched and will let the code calling Start Module.vi register for broadcasts and would permit the caller receive the broadcast that an error occurred at launch time."
      n126 = call-dynamic "Delacor_lib_QMH_Release Message Queue.vi"("error in"=w268, "Message Queue"=w261) -> ("error out"=w267:errorcluster)  [unwired: 9 in]
      n127 = call "Synchronize Caller Events.vi"("Singleton Module Admin in"=w262) -> ("error out"=w269:errorcluster)  [unwired: 9 in, 1 out]
      n128 = call "Module Name--constant.vi"() -> ("Module Name"=w265:string)  [unwired: 11 in]
      n129 = Format Into String(format string="An error occurred during initialization. %s is no longer running.", w265) -> (resulting string=w263:string)  [unwired: 2 in, 1 out]
      n130 = Merge Errors(w267, w269) -> (w270:errorcluster)
      n131 = call "Error Reported.vi"("Additional Information"=w263, "Error"=w270) -> ()  [unwired: 9 in, 1 out]
    }
  }
  n132 = Merge Errors(w17, w20) -> (w16:errorcluster)
  n133 = call "Close Module.vi"("error in"=w16, "Module Admin in"=w11) -> ("error out"=w18:errorcluster, "External Launch"=w4:bool, "Module Admin out"=w5:refnum<class "Delacor_lib_QMH_Module Admin.lvclass">)  [unwired: 7 in]
  n134 = Unregister For Events(event registration refnum=w10, error in=w18) -> (error out=w15:errorcluster)
  "error out" <- w15
  n135 = case "External Launch?" shown="False" w4 {
    tunnel: w15 -> [_ w271]
    frame False {
    }
    frame True {
      n136 = case shown="No Error" w271 {
        frame No Error {
          n137 = invoke on="Invoke Node" class="VI" method="FP.Close"() -> ()  [unwired: 3 in, 3 out]
        }
        frame Error {
          n138 = disable-structure shown="Default" {
            frame condition #0 (active) {
              n139 = invoke class="VI" method="FP.Open"("Activate"=TRUE ("Activate?")) -> ()  [unwired: 4 in, 5 out]
            }
            frame condition #1 {
              # "Don't show panel on error if running inside a built EXE."
            }
          }
        }
      }
    }
  }
  n140 = local write "Module Admin"(w5) -> ()
